vi "test_read-nmea-data2.vi"() -> ()   [LabVIEW 2019] (continued)
\n\t\n15:12:43.54\tF9P\t$GLGSV,2,1,08,69,12,031,,70,71,039,,71,52,205,28,72,04,209,,3*72\n\t\n15:12:43.56\tF9P\t$GLGSV,2,2,08,77,01,326,,84,20,122,,85,70,067,25,86,37,330,,3*7D\n\t\n15:12:43.58\tF9P\t$GAGSV,2,1,08,02,08,297,14,04,66,116,26,09,32,193,29,11,72,359,27,7*7A\n\t\n15:12:43.60\tF9P\t$GAGSV,2,2,08,12,40,103,26,19,26,045,15,25,09,249,,36,26,308,20,7*7A\n\t\n15:12:43.62\tF9P\t$GAGSV,2,1,08,02,08,297,,04,66,116,,09,32,193,35,11,72,359,,2*76\n\t\n15:12:43.64\tF9P\t$GAGSV,2,2,08,12,40,103,,19,26,045,,25,09,249,,36,26,308,,2*7D\n\t\n15:12:43.66\tF9P\t$GBGSV,1,1,04,11,50,132,32,14,87,127,30,28,,,42,33,60,219,42,1*4D\n\t\n15:12:43.68\tF9P\t$GBGSV,1,1,03,11,50,132,,14,87,127,28,33,60,219,,3*4A\n\t\n15:12:43.70\tF9P\t$GNGLL,3723.54718,N,12656.95403,E,061245.00,A,A*74\n\t\n15:12:43.72\tF9P\t\t\n15:12:43.74\tF9P\t\t\n15:12:43.76\tF9P\t\t\n15:12:43.78\tF9P\t\t\n15:12:43.80\tF9P\t\t\n15:12:43.82\tF9P\t\t\n15:12:43.84\tF9P\t\t\n15:12:43.86\tF9P\t\t\n15:12:43.88\tF9P\t\t\n15:12:43.90\tF9P\t\t\n15:12:43.92\tF9P\t\t\n15:12:43.94\tF9P\t\t\n15:12:43.96\tF9P\t\t\n15:12:43.98\tF9P\t\t\n15:12:44.00\tF9P\t\t\n15:12:44.02\tF9P\t\t\n15:12:44.04\tF9P\t\t\n15:12:44.06\tF9P\t\t\n15:12:44.08\tF9P\t\t\n15:12:44.10\tF9P\t\t\n15:12:44.12\tF9P\t\t\n15:12:44.14\tF9P\t\t\n15:12:44.16\tF9P\t\t\n15:12:44.18\tF9P\t\t\n15:12:44.20\tF9P\t\t\n15:12:44.22\tF9P\t\t\n15:12:44.24\tF9P\t$GNRMC,061246.00,A,3723.54779,N,12656.95458,E,2.347,47.63,250720,,,A,V*35\n\t\n15:12:44.26\tF9P\t$GNVTG,47.63,T,,M,2.347,N,4.346,K,A*12\n\t\n15:12:44.28\tF9P\t$GNGGA,061246.00,3723.54779,N,12656.95458,E,1,12,0.97,47.1,M,18.5,M,,*78\n\t\n15:12:44.30\tF9P\t$GNGSA,A,3,12,06,19,05,17,09,04,02,,,,,2.19,0.97,1.96,1*0A\n\t\n15:12:44.32\tF9P\t$GNGSA,A,3,85,70,71,84,,,,,,,,,2.19,0.97,1.96,2*08\n\t\n15:12:44.34\tF9P\t$GNGSA,A,3,36,19,11,04,09,12,,,,,,,2.19,0.97,1.96,3*0A\n\t\n15:12:44.36\tF9P\t$GNGSA,A,3,14,11,33,,,,,,,,,,2.19,0.97,1.96,4*0B\n\t\n15:12:44.38\tF9P\t$GPGSV,3,1,09,02,55,319,25,04,18,043,20,05,37,247,32,06,64,049,31,1*63\n\t\n15:12:44.40\tF9P\t$GPGSV,3,2,09,09,45,074,28,12,23,276,24,17,33,154,33,19,52,157,33,1*60\n\t\n15:12:44.42\tF9P\t$GPGSV,3,3,09,25,12,306,26,1*58\n\t\n15:12:44.44\tF9P\t$GPGSV,3,1,09,02,55,319,,04,18,043,17,05,37,247,24,06,64,049,26,6*66\n\t\n15:12:44.46\tF9P\t$GPGSV,3,2,09,09,45,074,29,12,23,276,,17,33,154,26,19,52,157,,6*64\n\t\n15:12:44.48\tF9P\t$GPGSV,3,3,09,25,12,306,22,6*5B\n\t\n15:12:44.50\tF9P\t$GLGSV,2,1,08,69,12,031,23,70,71,039,32,71,52,205,37,72,04,209,22,1*7E\n\t\n15:12:44.52\tF9P\t$GLGSV,2,2,08,77,01,326,,84,20,122,07,85,70,067,32,86,37,330,,1*7E\n\t\n15:12:44.54\tF9P\t$GLGSV,2,1,08,69,12,031,,70,71,039,,71,52,205,28,72,04,209,,3*72\n\t\n15:12:44.56\tF9P\t$GLGSV,2,2,08,77,01,326,,84,20,122,,85,70,067,25,86,37,330,,3*7D\n\t\n15:12:44.58\tF9P\t$GAGSV,2,1,08,02,08,297,11,04,66,116,26,09,32,193,34,11,72,359,27,7*73\n\t\n15:12:44.60\tF9P\t$GAGSV,2,2,08,12,40,103,27,19,26,045,15,25,09,249,,36,26,308,21,7*7A\n\t\n15:12:44.62\tF9P\t$GAGSV,2,1,08,02,08,297,,04,66,116,,09,32,193,,11,72,359,,2*70\n\t\n15:12:44.64\tF9P\t$GAGSV,2,2,08,12,40,103,,19,26,045,,25,09,249,,36,26,308,,2*7D\n\t\n15:12:44.66\tF9P\t$GBGSV,1,1,04,11,49,132,25,14,87,127,30,28,,,30,33,60,219,31,1*42\n\t\n15:12:44.68\tF9P\t$GBGSV,1,1,03,11,49,132,,14,87,127,,33,60,219,,3*48\n\t\n15:12:44.70\tF9P\t$GNGLL,3723.54779,N,12656.95458,E,061246.00,A,A*7E\n\t\n15:12:44.72\tF9P\t\t\n15:12:44.74\tF9P\t\t\n15:12:44.76\tF9P\t\t\n15:12:44.78\tF9P\t\t\n15:12:44.80\tF9P\t\t\n15:12:44.82\tF9P\t\t\n15:12:44.84\tF9P\t\t\n15:12:44.86\tF9P\t\t\n15:12:44.88\tF9P\t\t\n15:12:44.90\tF9P\t\t\n15:12:44.92\tF9P\t\t\n15:12:44.94\tF9P\t\t\n15:12:44.96\tF9P\t\t\n15:12:44.98\tF9P\t\t\n15:12:45.00\tF9P\t\t\n15:12:45.02\tF9P\t\t\n15:12:45.04\tF9P\t\t\n15:12:45.06\tF9P\t\t\n15:12:45.08\tF9P\t\t\n15:12:45.10\tF9P\t\t\n15:12:45.12\tF9P\t\t\n15:12:45.14\tF9P\t\t\n15:12:45.16\tF9P\t\t\n15:12:45.18\tF9P\t\t\n15:12:45.20\tF9P\t\t\n15:12:45.22\tF9P\t\t\n15:12:45.24\tF9P\t$GNRMC,061247.00,A,3723.54807,N,12656.95550,E,2.696,56.95,250720,,,A,V*3B\n\t\n15:12:45.26\tF9P\t$GNVTG,56.95,T,,M,2.696,N,4.993,K,A*10\n\t\n15:12:45.28\tF9P\t$GNGGA,061247.00,3723.54807,N,12656.95550,E,1,12,0.82,47.1,M,18.5,M,,*72\n\t\n15:12:45.30\tF9P\t$GNGSA,A,3,12,06,19,05,17,09,04,02,,,,,1.52,0.82,1.29,1*06\n\t\n15:12:45.32\tF9P\t$GNGSA,A,3,85,70,71,84,,,,,,,,,1.52,0.82,1.29,2*04\n\t\n15:12:45.34\tF9P\t$GNGSA,A,3,36,19,11,04,09,12,,,,,,,1.52,0.82,1.29,3*06\n\t\n15:12:45.36\tF9P\t$GNGSA,A,3,14,11,33,,,,,,,,,,1.52,0.82,1.29,4*07\n\t\n15:12:45.38\tF9P\t$GPGSV,3,1,09,02,55,319,31,04,18,043,22,05,37,247,38,06,64,049,26,1*68\n\t\n15:12:45.40\tF9P\t$GPGSV,3,2,09,09,45,074,28,12,23,276,23,17,33,154,32,19,52,157,29,1*6D\n\t\n15:12:45.42\tF9P\t$GPGSV,3,3,09,25,12,306,25,1*5B\n\t\n15:12:45.44\tF9P\t$GPGSV,3,1,09,02,55,319,,04,18,043,17,05,37,247,25,06,64,049,27,6*66\n\t\n15:12:45.46\tF9P\t$GPGSV,3,2,09,09,45,074,28,12,23,276,,17,33,154,26,19,52,157,,6*65\n\t\n15:12:45.48\tF9P\t$GPGSV,3,3,09,25,12,306,20,6*59\n\t\n15:12:45.50\tF9P\t$GLGSV,2,1,08,69,12,031,23,70,71,039,25,71,52,205,39,72,04,209,21,1*75\n\t\n15:12:45.52\tF9P\t$GLGSV,2,2,08,77,01,326,,84,20,122,12,85,70,067,32,86,37,330,,1*7A\n\t\n15:12:45.54\tF9P\t$GLGSV,2,1,08,69,12,031,,70,71,039,,71,52,205,27,72,04,209,,3*7D\n\t\n15:12:45.56\tF9P\t$GLGSV,2,2,08,77,01,326,,84,20,122,,85,70,067,23,86,37,330,,3*7B\n\t\n15:12:45.58\tF9P\t$GAGSV,2,1,08,02,08,297,09,04,66,116,25,09,32,193,28,11,72,359,27,7*74\n\t\n15:12:45.60\tF9P\t$GAGSV,2,2,08,12,40,103,28,19,26,045,17,25,09,249,,36,26,308,18,7*7D\n\t\n15:12:45.62\tF9P\t$GAGSV,2,1,08,02,08,297,,04,66,116,,09,32,193,,11,72,359,,2*70\n\t\n15:12:45.64\tF9P\t$GAGSV,2,2,08,12,40,103,,19,26,045,,25,09,249,,36,26,308,,2*7D\n\t\n15:12:45.66\tF9P\t$GBGSV,1,1,04,11,49,132,24,14,87,114,29,28,,,22,33,60,219,33,1*4A\n\t\n15:12:45.68\tF9P\t$GBGSV,1,1,03,11,49,132,,14,87,114,,33,60,219,,3*48\n\t\n15:12:45.70\tF9P\t$GNGLL,3723.54807,N,12656.95550,E,061247.00,A,A*70\n\t\n15:12:45.72\tF9P\t\t\n15:12:45.74\tF9P\t\t\n15:12:45.76\tF9P\t\t\n15:12:45.78\tF9P\t\t\n15:12:45.80\tF9P\t\t\n15:12:45.82\tF9P\t\t\n15:12:45.84\tF9P\t\t\n15:12:45.86\tF9P\t\t\n15:12:45.88\tF9P\t\t\n15:12:45.90\tF9P\t\t\n15:12:45.92\tF9P\t\t\n15:12:45.94\tF9P\t\t\n15:12:45.96\tF9P\t\t\n15:12:45.98\tF9P\t\t\n15:12:46.00\tF9P\t\t\n15:12:46.02\tF9P\t\t\n15:12:46.04\tF9P\t\t\n15:12:46.06\tF9P\t\t\n15:12:46.08\tF9P\t\t\n15:12:46.10\tF9P\t\t\n15:12:46.12\tF9P\t\t\n15:12:46.14\tF9P\t\t\n15:12:46.16\tF9P\t\t\n15:12:46.18\tF9P\t\t\n15:12:46.20\tF9P\t\t\n15:12:46.22\tF9P\t\t\n15:12:46.24\tF9P\t$GNRMC,061248.00,A,3723.54840,N,12656.95666,E,2.768,57.46,250720,,,A,V*3E\n\t\n15:12:46.26\tF9P\t$GNVTG,57.46,T,,M,2.768,N,5.126,K,A*18\n\t\n15:12:46.28\tF9P\t$GNGGA,061248.00,3723.54840,N,12656.95666,E,1,12,0.95,46.1,M,18.5,M,,*7F\n\t\n15:12:46.30\tF9P\t$GNGSA,A,3,12,06,19,05,17,09,04,02,,,,,1.88,0.95,1.62,1*08\n\t\n15:12:46.32\tF9P\t$GNGSA,A,3,85,70,71,84,,,,,,,,,1.88,0.95,1.62,2*0A\n\t\n15:12:46.34\tF9P\t$GNGSA,A,3,36,19,11,04,09,12,,,,,,,1.88,0.95,1.62,3*08\n\t\n15:12:46.36\tF9P\t$GNGSA,A,3,14,11,33,,,,,,,,,,1.88,0.95,1.62,4*09\n\t\n15:12:46.38\tF9P\t$GPGSV,3,1,09,02,55,319,27,04,18,043,24,05,37,247,43,06,64,049,31,1*63\n\t\n15:12:46.40\tF9P\t$GPGSV,3,2,09,09,45,074,32,12,23,276,29,17,33,154,37,19,52,157,29,1*69\n\t\n15:12:46.42\tF9P\t$GPGSV,3,3,09,25,12,306,24,1*5A\n\t\n15:12:46.44\tF9P\t$GPGSV,3,1,09,02,55,319,,04,18,043,17,05,37,247,25,06,64,049,27,6*66\n\t\n15:12:46.46\tF9P\t$GPGSV,3,2,09,09,45,074,27,12,23,276,,17,33,154,25,19,52,157,,6*69\n\t\n15:12:46.48\tF9P\t$GPGSV,3,3,09,25,12,306,16,6*5C\n\t\n15:12:46.50\tF9P\t$GLGSV,2,1,08,69,12,031,24,70,71,039,26,71,52,205,41,72,04,209,20,1*7F\n\t\n15:12:46.52\tF9P\t$GLGSV,2,2,08,77,01,326,,84,20,122,10,85,70,067,29,86,37,330,,1*72\n\t\n15:12:46.54\tF9P\t$GLGSV,2,1,08,69,12,031,,70,71,039,,71,52,205,31,72,04,209,,3*7A\n\t\n15:12:46.56\tF9P\t$GLGSV,2,2,08,77,01,326,,84,20,122,,85,70,067,21,86,37,330,,3*79\n\t\n15:12:46.58\tF9P\t$GAGSV,2,1,08,02,08,297,10,04,66,116,25,09,32,193,35,11,72,359,26,7*71\n\t\n15:12:46.60\tF9P\t$GAGSV,2,2,08,12,40,103,27,19,26,045,17,25,09,249,,36,26,308,21,7*78\n\t\n15:12:46.62\tF9P\t$GAGSV,2,1,08,02,08,297,,04,66,116,,09,32,193,,11,72,359,,2*70\n\t\n15:12:46.64\tF9P\t$GAGSV,2,2,08,12,40,103,,19,26,045,,25,09,249,,36,26,308,,2*7D\n\t\n15:12:46.66\tF9P\t$GBGSV,1,1,04,11,49,132,31,14,87,114,21,28,,,22,33,60,219,40,1*42\n\t\n15:12:46.68\tF9P\t$GBGSV,1,1,03,11,49,132,,14,87,114,,33,60,219,,3*48\n\t\n15:12:46.70\tF9P\t$GNGLL,3723.54840,N,12656.95666,E,061248.00,A,A*7A\n\t\n15:12:46.72\tF9P\t\t\n15:12:46.74\tF9P\t\t\n15:12:46.76\tF9P\t\t\n15:12:46.78\tF9P\t\t\n15:12:46.80\tF9P\t\t\n15:12:46.82\tF9P\t\t\n15:12:46.84\tF9P\t\t\n15:12:46.86\tF9P\t\t\n15:12:46.88\tF9P\t\t\n15:12:46.90\tF9P\t\t\n15:12:46.92\tF9P\t\t\n15:12:46.94\tF9P\t\t\n15:12:46.96\tF9P\t\t\n15:12:46.98\tF9P\t\t\n15:12:47.00\tF9P\t\t\n15:12:47.02\tF9P\t\t\n15:12:47.04\tF9P\t\t\n15:12:47.06\tF9P\t\t\n15:12:47.08\tF9P\t\t\n15:12:47.10\tF9P\t\t\n15:12:47.12\tF9P\t\t\n15:12:47.14\tF9P\t\t\n15:12:47.16\tF9P\t\t\n15:12:47.18\tF9P\t\t\n15:12:47.20\tF9P\t\t\n15:12:47.22\tF9P\t\t\n15:12:47.24\tF9P\t$GNRMC,061249.00,A,3723.54841,N,12656.95777,E,2.679,67.94,250720,,,A,V*32\n\t\n15:12:47.26\tF9P\t$GNVTG,67.94,T,,M,2.679,N,4.962,K,A*1C\n\t\n15:12:47.28\tF9P\t$GNGGA,061249.00,3723.54841,N,12656.95777,E,1,12,0.97,46.1,M,18.5,M,,*7C\n\t\n15:12:47.30\tF9P\t$GNGSA,A,3,12,06,19,05,17,09,04,02,,,,,2.19,0.97,1.96,1*0A\n\t\n15:12:47.32\tF9P\t$GNGSA,A,3,85,70,71,84,,,,,,,,,2.19,0.97,1.96,2*08\n\t\n15:12:47.34\tF9P\t$GNGSA,A,3,36,19,11,04,09,12,,,,,,,2.19,0.97,1.96,3*0A\n\t\n15:12:47.36\tF9P\t$GNGSA,A,3,14,11,33,,,,,,,,,,2.19,0.97,1.96,4*0B\n\t\n15:12:47.38\tF9P\t$GPGSV,3,1,09,02,55,319,30,04,18,043,23,05,37,247,41,06,64,049,31,1*60\n\t\n15:12:47.40\tF9P\t$GPGSV,3,2,09,09,45,074,33,12,23,276,29,17,33,154,28,19,52,157,35,1*6B\n\t\n15:12:47.42\tF9P\t$GPGSV,3,3,09,25,12,306,23,1*5D\n\t\n15:12:47.44\tF9P\t$GPGSV,3,1,09,02,55,319,,04,18,043,15,05,37,247,23,06,64,049,25,6*60\n\t\n15:12:47.46\tF9P\t$GPGSV,3,2,09,09,45,074,25,12,23,276,23,17,33,154,23,19,52,157,,6*6C\n\t\n15:12:47.48\tF9P\t$GPGSV,3,3,09,25,12,306,15,6*5F\n\t\n15:12:47.50\tF9P\t$GLGSV,2,1,08,69,12,031,24,70,71,039,27,71,52,205,39,72,04,209,21,1*70\n\t\n15:12:47.52\tF9P\t$GLGSV,2,2,08,77,01,326,,84,20,122,13,85,70,067,31,86,37,330,,1*78\n\t\n15:12:47.54\tF9P\t$GLGSV,2,1,08,69,12,031,21,70,71,039,,71,52,205,24,72,04,209,,3*7D\n\t\n15:12:47.56\tF9P\t$GLGSV,2,2,08,77,01,326,,84,20,122,,85,70,067,20,86,37,330,,3*78\n\t\n15:12:47.58\tF9P\t$GAGSV,2,1,08,02,08,297,10,04,66,116,26,09,32,193,34,11,72,359,27,7*72\n\t\n15:12:47.60\tF9P\t$GAGSV,2,2,08,12,40,103,32,19,26,045,17,25,09,249,,36,26,308,23,7*7E\n\t\n15:12:47.62\tF9P\t$GAGSV,2,1,08,02,08,297,,04,66,116,,09,32,193,,11,72,359,,2*70\n\t\n15:12:47.64\tF9P\t$GAGSV,2,2,08,12,40,103,,19,26,045,,25,09,249,,36,26,308,,2*7D\n\t\n15:12:47.66\tF9P\t$GBGSV,1,1,04,11,49,132,26,14,87,114,28,28,,,21,33,61,220,34,1*46\n\t\n15:12:47.68\tF9P\t$GBGSV,1,1,03,11,49,132,,14,87,114,26,33,61,220,,3*47\n\t\n15:12:47.70\tF9P\t$GNGLL,3723.54841,N,12656.95777,E,061249.00,A,A*7B\n\t\n15:12:47.72\tF9P\t\t\n15:12:47.74\tF9P\t\t\n15:12:47.76\tF9P\t\t\n15:12:47.78\tF9P\t\t\n15:12:47.80\tF9P\t\t\n15:12:47.82\tF9P\t\t\n15:12:47.84\tF9P\t\t\n15:12:47.86\tF9P\t\t\n15:12:47.88\tF9P\t\t\n15:12:47.90\tF9P\t\t\n15:12:47.92\tF9P\t\t\n15:12:47.94\tF9P\t\t\n15:12:47.96\tF9P\t\t\n15:12:47.98\tF9P\t\t\n15:12:48.00\tF9P\t\t\n15:12:48.02\tF9P\t\t\n15:12:48.04\tF9P\t\t\n15:12:48.06\tF9P\t\t\n15:12:48.08\tF9P\t\t\n15:12:48.10\tF9P\t\t\n15:12:48.12\tF9P\t\t\n15:12:48.14\tF9P\t\t\n15:12:48.16\tF9P\t\t\n15:12:48.18\tF9P\t\t\n15:12:48.20\tF9P\t\t\n15:12:48.22\tF9P\t\t\n15:12:48.24\tF9P\t$GNRMC,061250.00,A,3723.54855,N,12656.95833,E,1.133,52.99,250720,,,A,V*31\n\t\n15:12:48.26\tF9P\t$GNVTG,52.99,T,,M,1.133,N,2.099,K,A*16\n\t\n15:12:48.28\tF9P\t$GNGGA,061250.00,3723.54855,N,12656.95833,E,1,12,0.95,45.1,M,18.5,M,,*7F\n\t\n15:12:48.30\tF9P\t$GNGSA,A,3,12,06,19,05,17,09,04,02,,,,,1.88,0.95,1.62,1*08\n\t\n15:12:48.32\tF9P\t$GNGSA,A,3,85,70,71,84,,,,,,,,,1.88,0.95,1.62,2*0A\n\t\n15:12:48.34\tF9P\t$GNGSA,A,3,36,19,11,04,09,12,,,,,,,1.88,0.95,1.62,3*08\n\t\n15:12:48.36\tF9P\t$GNGSA,A,3,14,11,33,,,,,,,,,,1.88,0.95,1.62,4*09\n\t\n15:12:48.38\tF9P\t$GPGSV,3,1,09,02,55,319,26,04,18,043,22,05,37,247,40,06,64,049,31,1*67\n\t\n15:12:48.40\tF9P\t$GPGSV,3,2,09,09,45,074,30,12,23,276,21,17,33,154,28,19,52,157,36,1*63\n\t\n15:12:48.42\tF9P\t$GPGSV,3,3,09,25,12,306,24,1*5A\n\t\n15:12:48.44\tF9P\t$GPGSV,3,1,09,02,55,319,,04,18,043,16,05,37,247,22,06,64,049,25,6*62\n\t\n15:12:48.46\tF9P\t$GPGSV,3,2,09,09,45,074,27,12,23,276,22,17,33,154,21,19,52,157,,6*6D\n\t\n15:12:48.48\tF9P\t$GPGSV,3,3,09,25,12,306,17,6*5D\n\t\n15:12:48.50\tF9P\t$GLGSV,2,1,08,69,12,031,24,70,71,039,27,71,52,205,43,72,04,209,19,1*76\n\t\n15:12:48.52\tF9P\t$GLGSV,2,2,08,77,01,326,,84,20,122,11,85,70,067,26,86,37,330,,1*7C\n\t\n15:12:48.54\tF9P\t$GLGSV,2,1,08,69,12,031,20,70,71,039,,71,52,205,23,72,04,209,,3*7B\n\t\n15:12:48.56\tF9P\t$GLGSV,2,2,08,77,01,326,,84,20,122,,85,70,067,20,86,37,330,,3*78\n\t\n15:12:48.58\tF9P\t$GAGSV,2,1,08,02,08,297,26,04,66,116,27,09,32,193,41,11,72,359,28,7*7B\n\t\n15:12:48.60\tF9P\t$GAGSV,2,2,08,12,40,103,25,19,26,045,19,25,09,249,,36,26,308,29,7*7C\n\t\n15:12:48.62\tF9P\t$GAGSV,2,1,08,02,08,297,,04,66,116,,09,32,193,,11,72,359,,2*70\n\t\n15:12:48.64\tF9P\t$GAGSV,2,2,08,12,40,103,,19,26,045,,25,09,249,,36,26,308,,2*7D\n\t\n15:12:48.66\tF9P\t$GBGSV,1,1,04,11,49,132,31,14,87,114,27,28,,,33,33,61,220,37,1*4F\n\t\n15:12:48.68\tF9P\t$GBGSV,1,1,03,11,49,132,,14,87,114,25,33,61,220,,3*44\n\t\n15:12:48.70\tF9P\t$GNGLL,3723.54855,N,12656.95833,E,061250.00,A,A*79\n\t\n15:12:48.72\tF9P\t\t\n15:12:48.74\tF9P\t\t\n15:12:48.76\tF9P\t\t\n15:12:48.78\tF9P\t\t\n15:12:48.80\tF9P\t\t\n15:12:48.82\tF9P\t\t\n15:12:48.84\tF9P\t\t\n15:12:48.86\tF9P\t\t\n15:12:48.88\tF9P\t\t\n15:12:48.90\tF9P\t\t\n15:12:48.92\tF9P\t\t\n15:12:48.94\tF9P\t\t\n15:12:48.96\tF9P\t\t\n15:12:48.98\tF9P\t\t\n15:12:49.00\tF9P\t\t\n15:12:49.02\tF9P\t\t\n15:12:49.04\tF9P\t\t\n15:12:49.06\tF9P\t\t\n15:12:49.08\tF9P\t\t\n15:12:49.10\tF9P\t\t\n15:12:49.12\tF9P\t\t\n15:12:49.14\tF9P\t\t\n15:12:49.16\tF9P\t\t\n15:12:49.18\tF9P\t\t\n15:12:49.20\tF9P\t\t\n15:12:49.22\tF9P\t\t\n15:12:49.24\tF9P\t$GNRMC,061251.00,A,3723.54893,N,12656.95891,E,2.233,52.49,250720,,,A,V*3F\n\t\n15:12:49.26\tF9P\t$GNVTG,52.49,T,,M,2.233,N,4.135,K,A*1A\n\t\n15:12:49.28\tF9P\t$GNGGA,061251.00,3723.54893,N,12656.95891,E,1,12,0.95,44.7,M,18.5,M,,*7B\n\t\n15:12:49.30\tF9P\t$GNGSA,A,3,12,06,19,05,17,09,04,02,,,,,1.88,0.95,1.62,1*08\n\t\n15:12:49.32\tF9P\t$GNGSA,A,3,85,70,71,84,,,,,,,,,1.88,0.95,1.62,2*0A\n\t\n15:12:49.34\tF9P\t$GNGSA,A,3,36,19,11,04,09,12,,,,,,,1.88,0.95,1.62,3*08\n\t\n15:12:49.36\tF9P\t$GNGSA,A,3,14,11,33,,,,,,,,,,1.88,0.95,1.62,4*09\n\t\n15:12:49.38\tF9P\t$GPGSV,3,1,09,02,55,319,27,04,18,043,24,05,37,247,40,06,64,049,26,1*66\n\t\n15:12:49.40\tF9P\t$GPGSV,3,2,09,09,45,074,32,12,23,276,28,17,33,154,34,19,52,157,27,1*65\n\t\n15:12:49.42\tF9P\t$GPGSV,3,3,09,25,12,306,25,1*5B\n\t\n15:12:49.44\tF9P\t$GPGSV,3,1,09,02,55,319,,04,18,043,18,05,37,247,23,06,64,049,22,6*6A\n\t\n15:12:49.46\tF9P\t$GPGSV,3,2,09,09,45,074,27,12,23,276,21,17,33,154,19,19,52,157,,6*65\n\t\n15:12:49.48\tF9P\t$GPGSV,3,3,09,25,12,306,19,6*53\n\t\n15:12:49.50\tF9P\t$GLGSV,2,1,08,69,12,031,24,70,71,039,27,71,52,205,39,72,04,209,20,1*71\n\t\n15:12:49.52\tF9P\t$GLGSV,2,2,08,77,01,326,,84,20,122,12,85,70,067,31,86,37,330,,1*79\n\t\n15:12:49.54\tF9P\t$GLGSV,2,1,08,69,12,031,20,70,71,039,,71,52,205,22,72,04,209,,3*7A\n\t\n15:12:49.56\tF9P\t$GLGSV,2,2,08,77,01,326,,84,20,122,,85,70,067,20,86,37,330,,3*78\n\t\n15:12:49.58\tF9P\t$GAGSV,2,1,08,02,08,297,29,04,66,116,26,09,32,193,34,11,72,359,29,7*76\n\t\n15:12:49.60\tF9P\t$GAGSV,2,2,08,12,40,103,26,19,26,045,19,25,09,249,,36,26,308,21,7*77\n\t\n15:12:49.62\tF9P\t$GAGSV,2,1,08,02,08,297,,04,66,116,,09,32,193,,11,72,359,,2*70\n\t\n15:12:49.64\tF9P\t$GAGSV,2,2,08,12,40,103,,19,26,045,,25,09,249,,36,26,308,,2*7D\n\t\n15:12:49.66\tF9P\t$GBGSV,1,1,04,11,49,132,31,14,87,114,28,28,,,29,33,61,220,32,1*4E\n\t\n15:12:49.68\tF9P\t$GBGSV,1,1,03,11,49,132,,14,87,114,,33,61,220,,3*43\n\t\n15:12:49.70\tF9P\t$GNGLL,3723.54893,N,12656.95891,E,061251.00,A,A*7A\n\t\n15:12:49.72\tF9P\t\t\n15:12:49.74\tF9P\t\t\n15:12:49.76\tF9P\t\t\n15:12:49.78\tF9P\t\t\n15:12:49.80\tF9P\t\t\n15:12:49.82\tF9P\t\t\n15:12:49.84\tF9P\t\t\n15:12:49.86\tF9P\t\t\n15:12:49.88\tF9P\t\t\n15:12:49.90\tF9P\t\t\n15:12:49.92\tF9P\t\t\n15:12:49.94\tF9P\t\t\n15:12:49.96\tF9P\t\t\n15:12:49.98\tF9P\t\t\n15:12:50.00\tF9P\t\t\n15:12:50.02\tF9P\t\t\n15:12:50.04\tF9P\t\t\n15:12:50.06\tF9P\t\t\n15:12:50.08\tF9P\t\t\n15:12:50.10\tF9P\t\t\n15:12:50.12\tF9P\t\t\n15:12:50.14\tF9P\t\t\n15:12:50.16\tF9P\t\t\n15:12:50.18\tF9P\t\t\n15:12:50.20\tF9P\t\t\n15:12:50.22\tF9P\t\t\n15:12:50.24\tF9P\t$GNRMC,061252.00,A,3723.54901,N,12656.95976,E,2.427,62.78,250720,,,A,V*3C\n\t\n15:12:50.26\tF9P\t$GNVTG,62.78,T,,M,2.427,N,4.495,K,A*17\n\t\n15:12:50.28\tF9P\t$GNGGA,061252.00,3723.54901,N,12656.95976,E,1,12,0.95,45.2,M,18.5,M,,*7E\n\t\n15:12:50.30\tF9P\t$GNGSA,A,3,12,06,19,05,17,09,04,02,,,,,1.88,0.95,1.62,1*08\n\t\n15:12:50.32\tF9P\t$GNGSA,A,3,85,70,71,84,,,,,,,,,1.88,0.95,1.62,2*0A\n\t\n15:12:50.34\tF9P\t$GNGSA,A,3,36,19,11,04,09,12,,,,,,,1.88,0.95,1.62,3*08\n\t\n15:12:50.36\tF9P\t$GNGSA,A,3,14,11,33,,,,,,,,,,1.88,0.95,1.62,4*09\n\t\n15:12:50.38\tF9P\t$GPGSV,3,1,09,02,55,319,25,04,18,043,25,05,37,247,42,06,64,049,26,1*67\n\t\n15:12:50.40\tF9P\t$GPGSV,3,2,09,09,45,074,30,12,23,276,32,17,33,154,29,19,52,157,28,1*6F\n\t\n15:12:50.42\tF9P\t$GPGSV,3,3,09,25,12,306,30,1*5F\n\t\n15:12:50.44\tF9P\t$GPGSV,3,1,09,02,55,319,,04,18,043,19,05,37,247,24,06,64,049,23,6*6D\n\t\n15:12:50.46\tF9P\t$GPGSV,3,2,09,09,45,074,27,12,23,276,21,17,33,154,17,19,52,157,,6*6B\n\t\n15:12:50.48\tF9P\t$GPGSV,3,3,09,25,12,306,20,6*59\n\t\n15:12:50.50\tF9P\t$GLGSV,2,1,08,69,12,031,25,70,71,039,26,71,52,205,43,72,04,209,21,1*7D\n\t\n15:12:50.52\tF9P\t$GLGSV,2,2,08,77,01,326,,84,20,122,11,85,70,067,27,86,37,330,,1*7D\n\t\n15:12:50.54\tF9P\t$GLGSV,2,1,08,69,12,031,18,70,71,039,,71,52,205,30,72,04,209,,3*72\n\t\n15:12:50.56\tF9P\t$GLGSV,2,2,08,77,01,326,,84,20,122,,85,70,067,21,86,37,330,,3*79\n\t\n15:12:50.58\tF9P\t$GAGSV,2,1,08,02,08,297,19,04,66,116,26,09,32,193,38,11,72,359,29,7*79\n\t\n15:12:50.60\tF9P\t$GAGSV,2,2,08,12,40,103,29,19,26,045,20,25,09,249,,36,26,308,23,7*70\n\t\n15:12:50.62\tF9P\t$GAGSV,2,1,08,02,08,297,,04,66,116,,09,32,193,,11,72,359,,2*70\n\t\n15:12:50.64\tF9P\t$GAGSV,2,2,08,12,40,103,,19,26,045,,25,09,249,,36,26,308,,2*7D\n\t\n15:12:50.66\tF9P\t$GBGSV,1,1,04,11,49,132,30,14,87,114,27,28,,,22,33,61,220,38,1*41\n\t\n15:12:50.68\tF9P\t$GBGSV,1,1,04,10,,,33,11,49,132,,14,87,114,,33,61,220,,3*45\n\t\n15:12:50.70\tF9P\t$GNGLL,3723.54901,N,12656.95976,E,061252.00,A,A*7B\n\t\n15:12:50.72\tF9P\t\t\n15:12:50.74\tF9P\t\t\n15:12:50.76\tF9P\t\t\n15:12:50.78\tF9P\t\t\n15:12:50.80\tF9P\t\t\n15:12:50.82\tF9P\t\t\n15:12:50.84\tF9P\t\t\n15:12:50.86\tF9P\t\t\n15:12:50.88\tF9P\t\t\n15:12:50.90\tF9P\t\t\n15:12:50.92\tF9P\t\t\n15:12:50.94\tF9P\t\t\n15:12:50.96\tF9P\t\t\n15:12:50.98\tF9P\t\t\n15:12:51.00\tF9P\t\t\n15:12:51.02\tF9P\t\t\n15:12:51.04\tF9P\t\t\n15:12:51.06\tF9P\t\t\n15:12:51.08\tF9P\t\t\n15:12:51.10\tF9P\t\t\n15:12:51.12\tF9P\t\t\n15:12:51.14\tF9P\t\t\n15:12:51.16\tF9P\t\t\n15:12:51.18\tF9P\t\t\n15:12:51.20\tF9P\t\t\n15:12:51.22\tF9P\t\t\n15:12:51.24\tF9P\t$GNRMC,061253.00,A,3723.54935,N,12656.96073,E,2.562,63.38,250720,,,A,V*30\n\t\n15:12:51.26\tF9P\t$GNVTG,63.38,T,,M,2.562,N,4.744,K,A*1D\n\t\n15:12:51.28\tF9P\t$GNGGA,061253.00,3723.54935,N,12656.96073,E,1,12,0.83,44.7,M,18.5,M,,*74\n\t\n15:12:51.30\tF9P\t$GNGSA,A,3,12,06,19,05,17,09,04,02,,,,,1.56,0.83,1.32,1*09\n\t\n15:12:51.32\tF9P\t$GNGSA,A,3,85,70,71,84,,,,,,,,,1.56,0.83,1.32,2*0B\n\t\n15:12:51.34\tF9P\t$GNGSA,A,3,36,19,11,04,09,12,,,,,,,1.56,0.83,1.32,3*09\n\t\n15:12:51.36\tF9P\t$GNGSA,A,3,14,11,33,,,,,,,,,,1.56,0.83,1.32,4*08\n\t\n15:12:51.38\tF9P\t$GPGSV,3,1,09,02,55,319,23,04,18,043,25,05,37,247,32,06,
